vi "serial-read-subVi.vi"(8 "error in":errorcluster, 10 "state":string="init", 11 "VISA resource name":refnum<visa-resource-name>="COM22") -> (0 "error out":errorcluster, 1 "read buffer out":string, 2 "all-sensor-data":T4 {"dP3"."Temp (degC)" format="%.2f"; "dP3"."dP (mBar)" format="%.2f"; "dP2"."Temp (degC)" format="%.2f"; "dP2"."dP (mBar)" format="%.2f"; "dP1"."Temp (degC)" format="%.2f"; "dP1"."dP (mBar)" format="%.2f"; "CD4"."CO2 (ppm)" format="%.2f"; "CD3"."CO2 (ppm)" format="%.2f"; "RHT4"."Humidity (%)" format="%.2f"; "RHT4"."Temp (degC)" format="%.2f"; "RHT5"."Humidity (%)" format="%.2f"; "RHT5"."Temp (degC)" format="%.2f"; "CD2"."Humidity (%)" format="%.2f"; "CD2"."Temp (degC)" format="%.2f"; "CD2"."CO2 (ppm)" format="%.2f"; "RHT3"."Humidity (%)" format="%.2f"; "RHT3"."Temp (degC)" format="%.2f"; "CD6"."CO2 (ppm)" format="%.2f"; "RHT6"."Humidity (%)" format="%.2f"; "RHT6"."Temp (degC)" format="%.2f"; "CD5"."CO2 (ppm)" format="%.2f"; "CD1"."Humidity (%)" format="%.2f"; "CD1"."Temp (degC)" format="%.2f"; "CD1"."CO2 (ppm)" format="%.2f"}, 3 "VISA resource out":refnum<visa-resource-name>)   [LabVIEW 2021]
uses:
  all-sensor-data.ctl
  SCD41.ctl
  STC31.ctl
  SHT41.ctl
  SDP810.ctl
  <vilib>/Instr/_visa.llb/VISA Configure Serial Port (Instr).vi
panel:
  out "x > y?":bool
  out "RHT4":T1 {"Humidity (%)" format="%.2f"; "Temp (degC)" format="%.2f"}
  out "RHT3":T1 {"Humidity (%)" format="%.2f"; "Temp (degC)" format="%.2f"}
  out "RHT6":T1 {"Humidity (%)" format="%.2f"; "Temp (degC)" format="%.2f"}
  out "RHT5":T1 {"Humidity (%)" format="%.2f"; "Temp (degC)" format="%.2f"}
  out "CD6":T2 {"CO2 (ppm)" format="%.2f"}
  out "CD5":T2 {"CO2 (ppm)" format="%.2f"}
  out "CD4":T2 {"CO2 (ppm)" format="%.2f"}
  out "CD3":T2 {"CO2 (ppm)" format="%.2f"}
  out "CD2":T3 {"Humidity (%)" format="%.2f"; "Temp (degC)" format="%.2f"; "CO2 (ppm)" format="%.2f"}
  out "CD1":T3 {"Humidity (%)" format="%.2f"; "Temp (degC)" format="%.2f"; "CO2 (ppm)" format="%.2f"}
  out "Num Samples":i32
  out "data string array":string[](array[string])
  out "read buffer":string
  out "Bytes Returned":u32
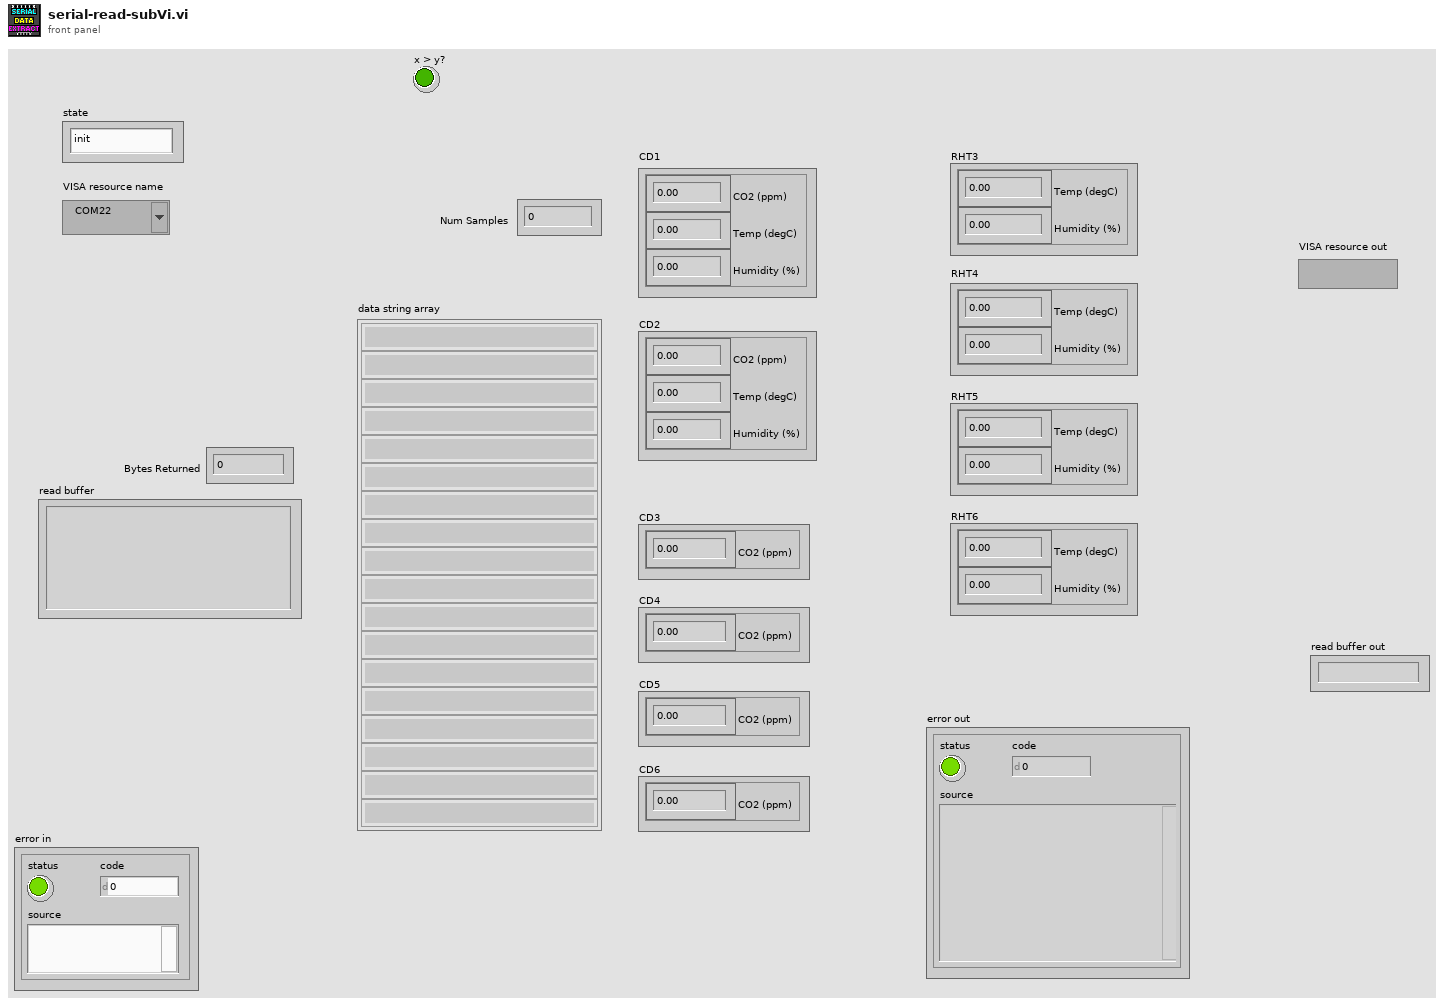
[diagram p1: front panel]
types:
  T1 = typedef "SHT41.ctl" = cluster{"Temp (degC)":dbl, "Humidity (%)":dbl}
  T2 = typedef "STC31.ctl" = cluster{"CO2 (ppm)":dbl}
  T3 = typedef "SCD41.ctl" = cluster{"CO2 (ppm)":dbl, "Temp (degC)":dbl, "Humidity (%)":dbl}
  T4 = typedef "all-sensor-data.ctl" = cluster{"CD1":T3, "CD2":T3, "CD3":T2, "CD4":T2, "CD5":T2, "CD6":T2, "RHT3":T1, "RHT4":T1, "RHT5":T1, "RHT6":T1, "dP1":T5, "dP2":T5, "dP3":T5}
  T5 = typedef "SDP810.ctl" = cluster{"dP (mBar)":dbl, "Temp (degC)":dbl}
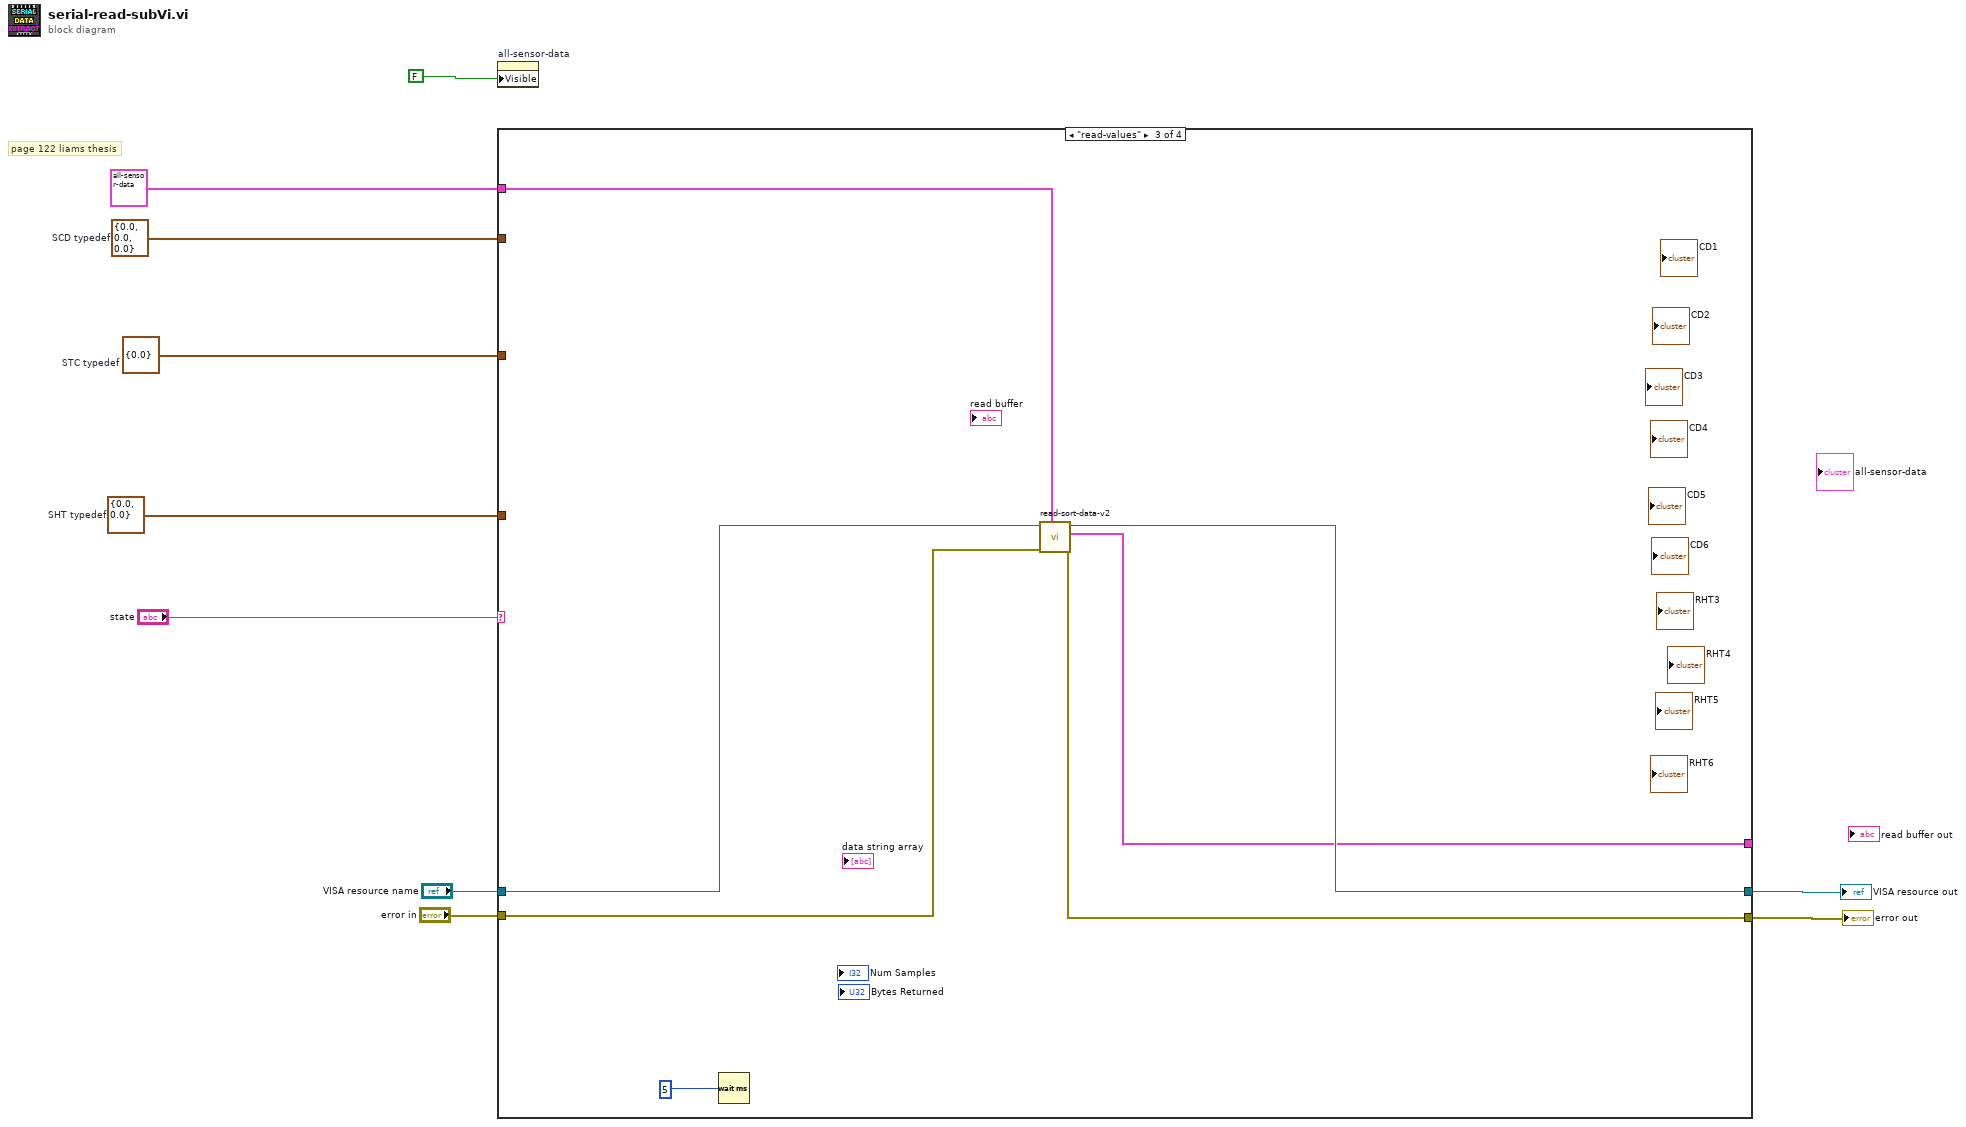
[diagram p0: block diagram]
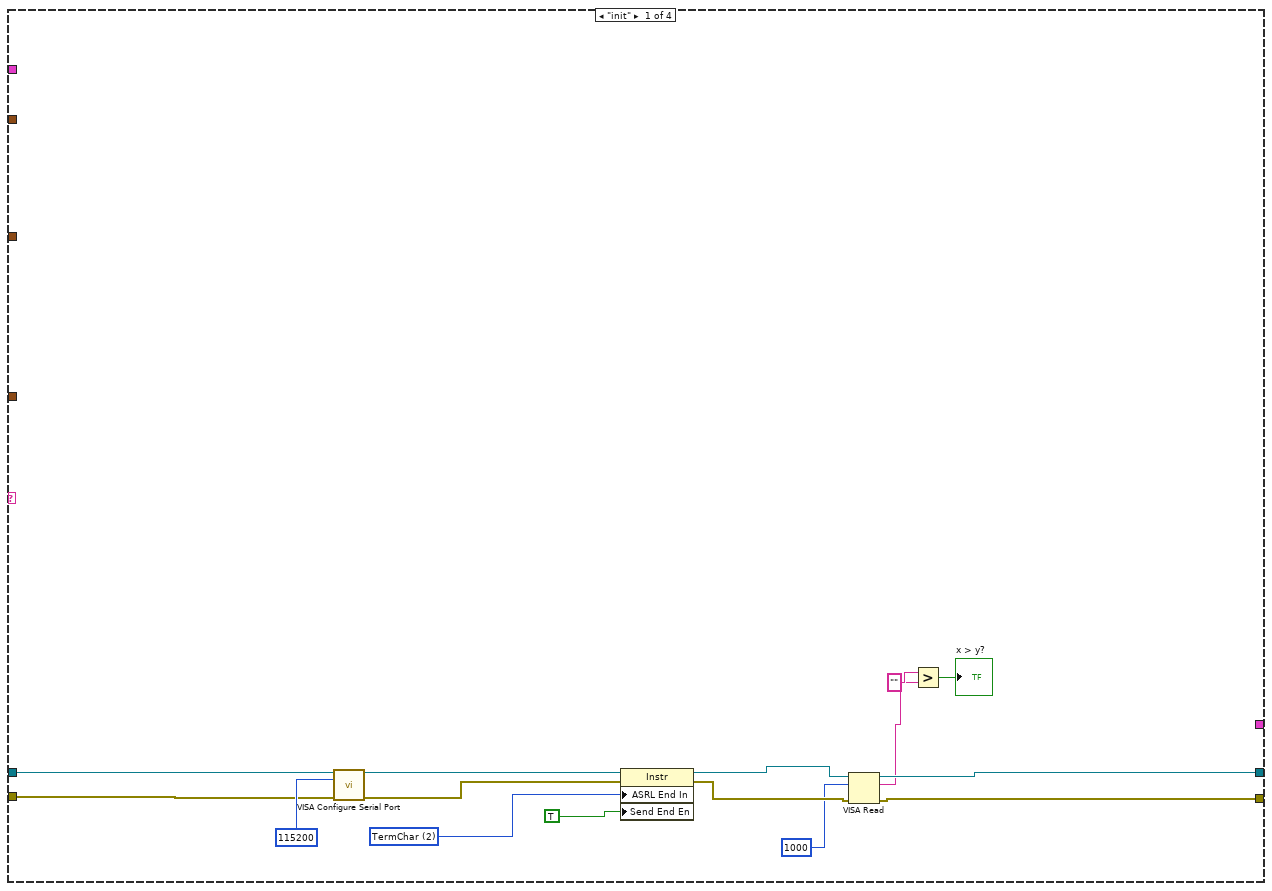
[diagram p2: hidden frame]
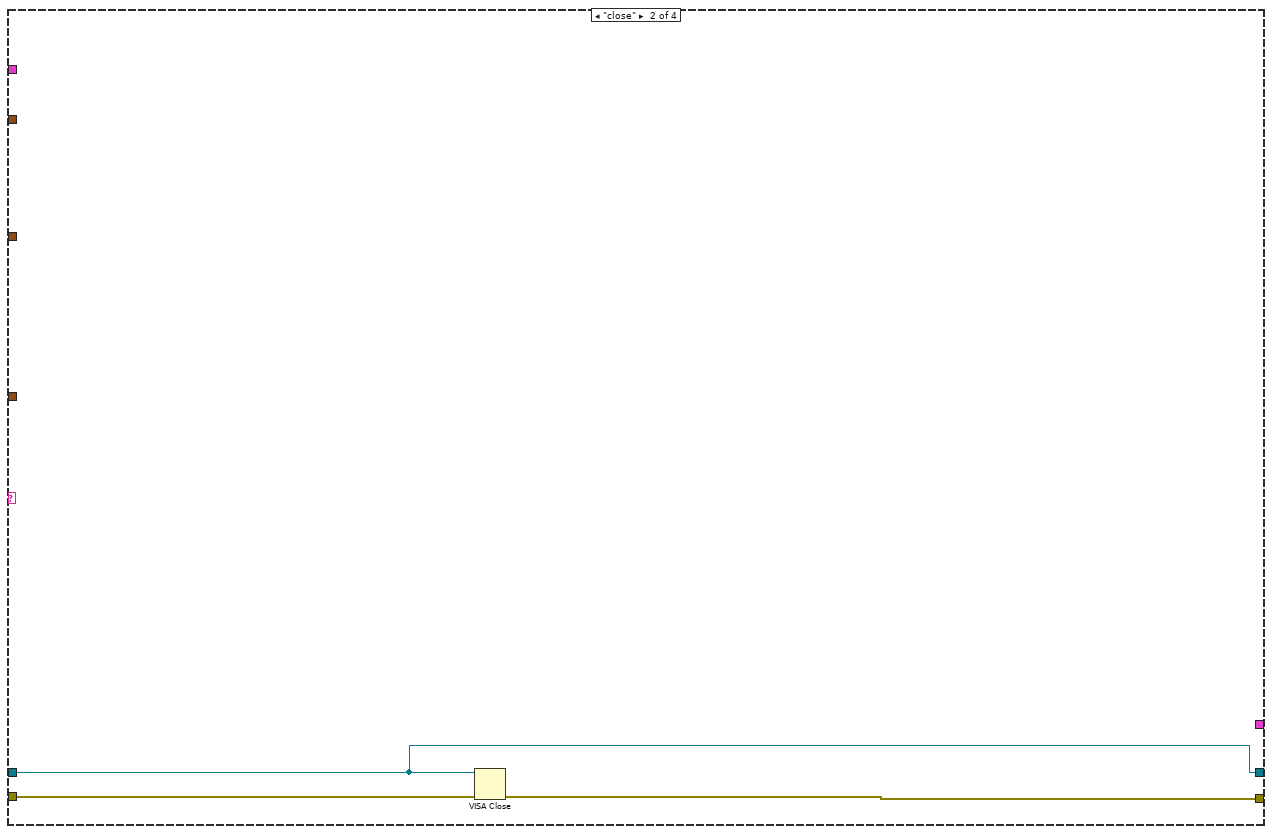
[diagram p3: hidden frame]
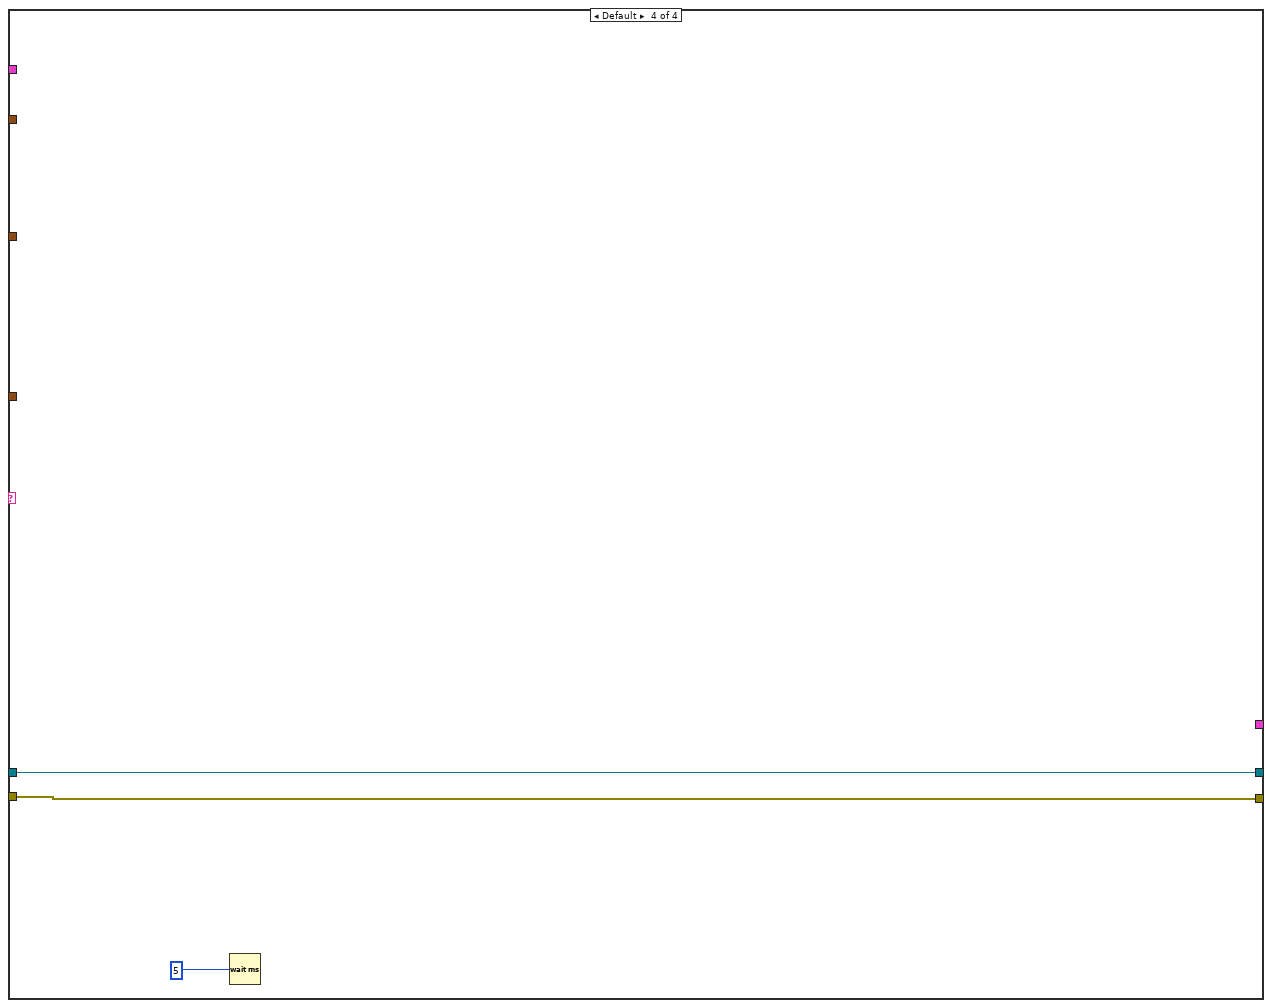
[diagram p4: hidden frame]
diagram:
  w6 = T1 {"Temp (degC)"=0.0, "Humidity (%)"=0.0}  # SHT typedef
  w7 = T2 {"CO2 (ppm)"=0.0}  # STC typedef
  w8 = T3 {"CO2 (ppm)"=0.0, "Temp (degC)"=0.0, "Humidity (%)"=0.0}  # SCD typedef
  # "page 122 liams thesis"
  n1 = property on="all-sensor-data" class="Clust (strict)"("Visible"=FALSE) -> ()  [unwired: 2 in, 2 out]
  n2 = case shown="\"read-values\"" "state" {
    tunnel: "VISA resource name" -> [w20 w26 w34 w37]
    tunnel: w8 -> [_ _ _ _]
    tunnel: w7 -> [_ _ _ _]
    tunnel: w6 -> [_ _ _ _]
    tunnel: T4 {"CD1"={"CO2 (ppm)"=0.0, "Temp (degC)"=0.0, "Humidity (%)"=0.0}, "CD2"={"CO2 (ppm)"=0.0, "Temp (degC)"=0.0, "Humidity (%)"=0.0}, "CD3"={"CO2 (ppm)"=0.0}, "CD4"={"CO2 (ppm)"=0.0}, "CD5"={"CO2 (ppm)"=0.0}, "CD6"={"CO2 (ppm)"=0.0}, "RHT3"={"Temp (degC)"=0.0, "Humidity (%)"=0.0}, "RHT4"={"Temp (degC)"=0.0, "Humidity (%)"=0.0}, "RHT5"={"Temp (degC)"=0.0, "Humidity (%)"=0.0}, "RHT6"={"Temp (degC)"=0.0, "Humidity (%)"=0.0}, "dP1"={"dP (mBar)"=0.0, "Temp (degC)"=0.0}, "dP2"={"dP (mBar)"=0.0, "Temp (degC)"=0.0}, "dP3"={"dP (mBar)"=0.0, "Temp (degC)"=0.0}} ("all-data") -> [_ _ w29 _]
    tunnel: "error in" -> [w19 w28 w33 w36]
    tunnel: [w15 w27 w31 w36] -> w3
    tunnel: [w17 w26 w32 w37] -> w2
    tunnel: [_ _ w30 _] -> _
    frame "init" {
      w23 = u16 2 items=["None", "Last Bit", "TermChar"] ("Serial Settings:End Mode for Reads")
      n3 = call-poly "VISA Configure Serial Port"("VISA resource name"=w20, "baud rate (9600)"=u32 115200, "error in (no error)"=w19) -> ("VISA resource name out"=w24:refnum<visa-resource-name>, "error out"=w25:errorcluster)  [unwired: 11 in]
      n4 = property class="Instr"(reference=w24, error in=w25, "ASRL End In"=w23, "Send End En"=TRUE ("Message Based Settings:Send End Enable")) -> (reference out=w18:refnum<visa-resource-name>, error out=w16:errorcluster)
      n5 = VISA Read(VISA resource name=w18, byte count=u32 1000, error in (no error)=w16) -> (VISA resource name out=w17:refnum<visa-resource-name>, read buffer=w14:string, error out=w15:errorcluster)  [unwired: 1 out]
      n6 = Greater?(x=w14, y="") -> (0:→"x > y?":bool)
    }
    frame "close" {
      n7 = VISA Close(VISA resource name=w26, error in (no error)=w28) -> (error out=w27:errorcluster)
    }
    frame "read-values" {
      n8 = Wait (ms)(milliseconds to wait=u32 5) -> ()  [unwired: 1 out]
      n9 = call "read-sort-data-v2.vi"("all-data in"=w29, "error in (no error)"=w33, "VISA Refnum in"=w34) -> ("error out"=w31:errorcluster, "all-data out"=w30:T4, "VISA Refnum out"=w32:refnum<visa-resource-name>)  [unwired: 4 in, 2 out]
    }
    frame Default {
      n10 = Wait (ms)(milliseconds to wait=u32 5) -> ()  [unwired: 1 out]
    }
  }
  "error out" <- w3
  "VISA resource out" <- w2
